vi "Get OOB Server Address.vi"() -> (0 "error out":errorcluster, 3 "Address":string)   [LabVIEW 2026]
panel:
  out "Ports":u16[](array[numeric])
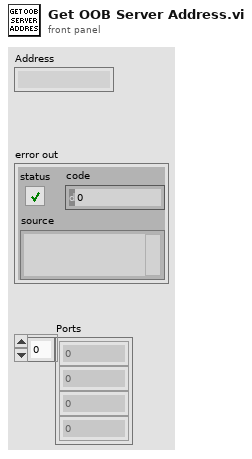
[diagram p1: front panel]
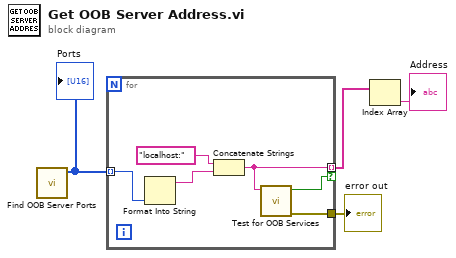
[diagram p0: block diagram]
diagram:
  n1 = call "Find OOB Server Ports.vi"() -> ("Ports"=w4:u16[])  [unwired: 11 in]
  "Ports" <- w4
  n2 = for {
    tunnel: [w8] -> w2 mode=indexing if=w6
    tunnel: w4 -> [w7] mode=indexing
    tunnel: [w5] -> w3
    n3 = Format Into String(w7) -> (resulting string=w10:string)  [unwired: 3 in, 1 out]
    n4 = Concatenate Strings("localhost:" ("string"), w10) -> (w8:string)
    n5 = call "Test for OOB Services.vi"("address"=w8) -> ("error out"=w5:errorcluster, "Found OOB Server"=w6:bool)  [unwired: 9 in]
  }
  "error out" <- w3
  n6 = Index Array(array=w2) -> (element=→"Address":string)  [unwired: 1 in]
